vi "StartupGISErrorMonitor.vi"(8 "error in (no error)":errorcluster, 10 "GIS Printer":refnum<class "GIS Printer.lvclass">, 11 "TopLevel in":refnum<class "TopLevel.lvclass">) -> (0 "error out":errorcluster)   [LabVIEW 2022 SP3, in "GIS Printer.lvclass"]
uses:
  GIS Printer.lvclass
  TopLevel/TopLevel.lvclass
  GIS Error Monitor Process.vi
panel:
  out "timed out?":bool
  out "sync from process?":bool
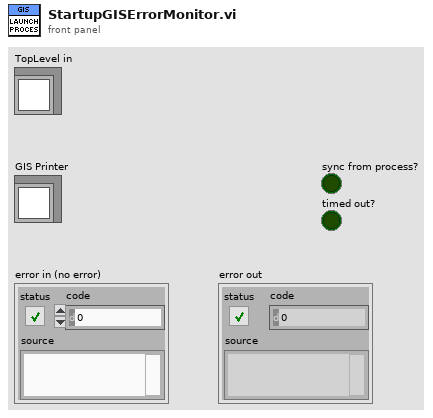
[diagram p1: front panel]
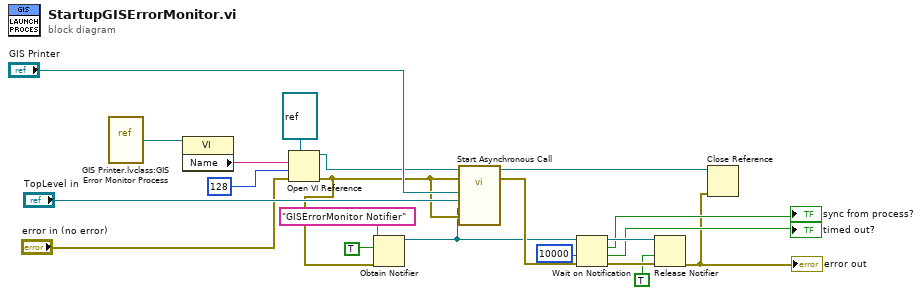
[diagram p0: block diagram]
diagram:
  n1 = vi-ref "GIS Printer.lvclass:GIS Error Monitor Process.vi"() -> (w13:refnum<vi>)
  n2 = property class="VI"(reference=w13) -> ("Name"=w14:string)  [unwired: 1 in, 2 out]
  n3 = Open VI Reference(type specifier VI Refnum (for type only)=refnum<vi> refnum, vi path=w14, options=128, error in (no error)="error in (no error)") -> (vi reference=w16:refnum<vi>, error out=w10:errorcluster)  [unwired: 2 in]
  n4 = Obtain Notifier(name (unnamed)="GISErrorMonitor Notifier", notification data type=TRUE, error in (no error)=w10) -> (notifier out=w1:refnum<notifier>)  [unwired: 1 in, 2 out]
  n5 = call-by-ref "Start Asynchronous Call"(reference=w16, error in=w10, "error in"=w10, "notifierSync"=w1, "TopLevel"="TopLevel in", "GIS Printer in"="GIS Printer") -> (reference out=w17:refnum<vi>, error out=w3:errorcluster)  [unwired: 7 in, 1 out]
  n6 = Wait on Notification(notifier=w1, timeout in ms (-1)=10000, error in (no error)=w3) -> (notifier out=w7:refnum<notifier>, notification=→"sync from process?":bool, timed out?=→"timed out?":bool, error out=w8:errorcluster)  [unwired: 1 in]
  n7 = Release Notifier(notifier=w7, force destroy? (F)=TRUE, error in (no error)=w8) -> (error out=w2:errorcluster)  [unwired: 2 out]
  "error out" <- w2
  n8 = Close Reference(reference=w17, error in (no error)=w2) -> ()  [unwired: 1 out]
